vi "24 Global Front Panel (2017).vi"() -> ()   [LabVIEW 2017]
panel:
  out "Id_scale":dbl
  out "Ic_scale":dbl
  out "Ib_scale":dbl
  out "Ia_scale":dbl
  out "Vd_scale":dbl
  out "Vc_scale":dbl
  out "Vb_scale":dbl
  out "Va_Scale":dbl
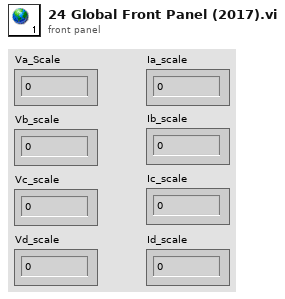
[diagram p1: front panel]
diagram:
